vi "Understanding DataFlow.vi"() -> ()   [LabVIEW 2026]
panel:
  out "Thermometer (C)":dbl(slide) scale=0.0..100.0
  in  "Temperature (F)":dbl(slide) scale=0.0..200.0
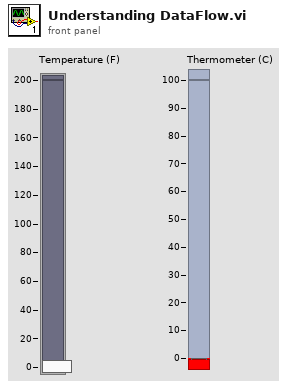
[diagram p1: front panel]
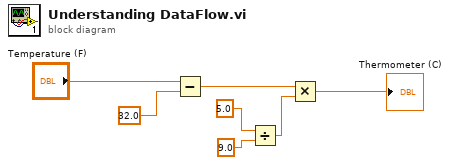
[diagram p0: block diagram]
diagram:
  n1 = Subtract(x="Temperature (F)", y=32.0) -> (x-y=w3:dbl)
  n2 = Divide(x=5.0, y=9.0) -> (x/y=w2:dbl)
  n3 = Multiply(x=w3, y=w2) -> (x*y=→"Thermometer (C)":dbl)
